vi "Untitled 1.vi"() -> ()   [LabVIEW 2026]
uses:
  CaptureJSONtypedef.ctl
  35900ef4-9114-49d9-b2d4-e1f00d13cbe6.vi
  <vilib>/JDP Science/JSONtext/JSON text to Variant.vi
  <vilib>/JDP Science/JSONtext/LVClass Serializer/JSONtext LVClass Serializer.lvclass
panel:
  out "Delta tMs":i32[](array[numeric])
  out "timingTicks64":string[](array[string])
  out "tMs":i32[](array[numeric])
  out "Index":i32[](array[numeric])
  out "Data out":T1
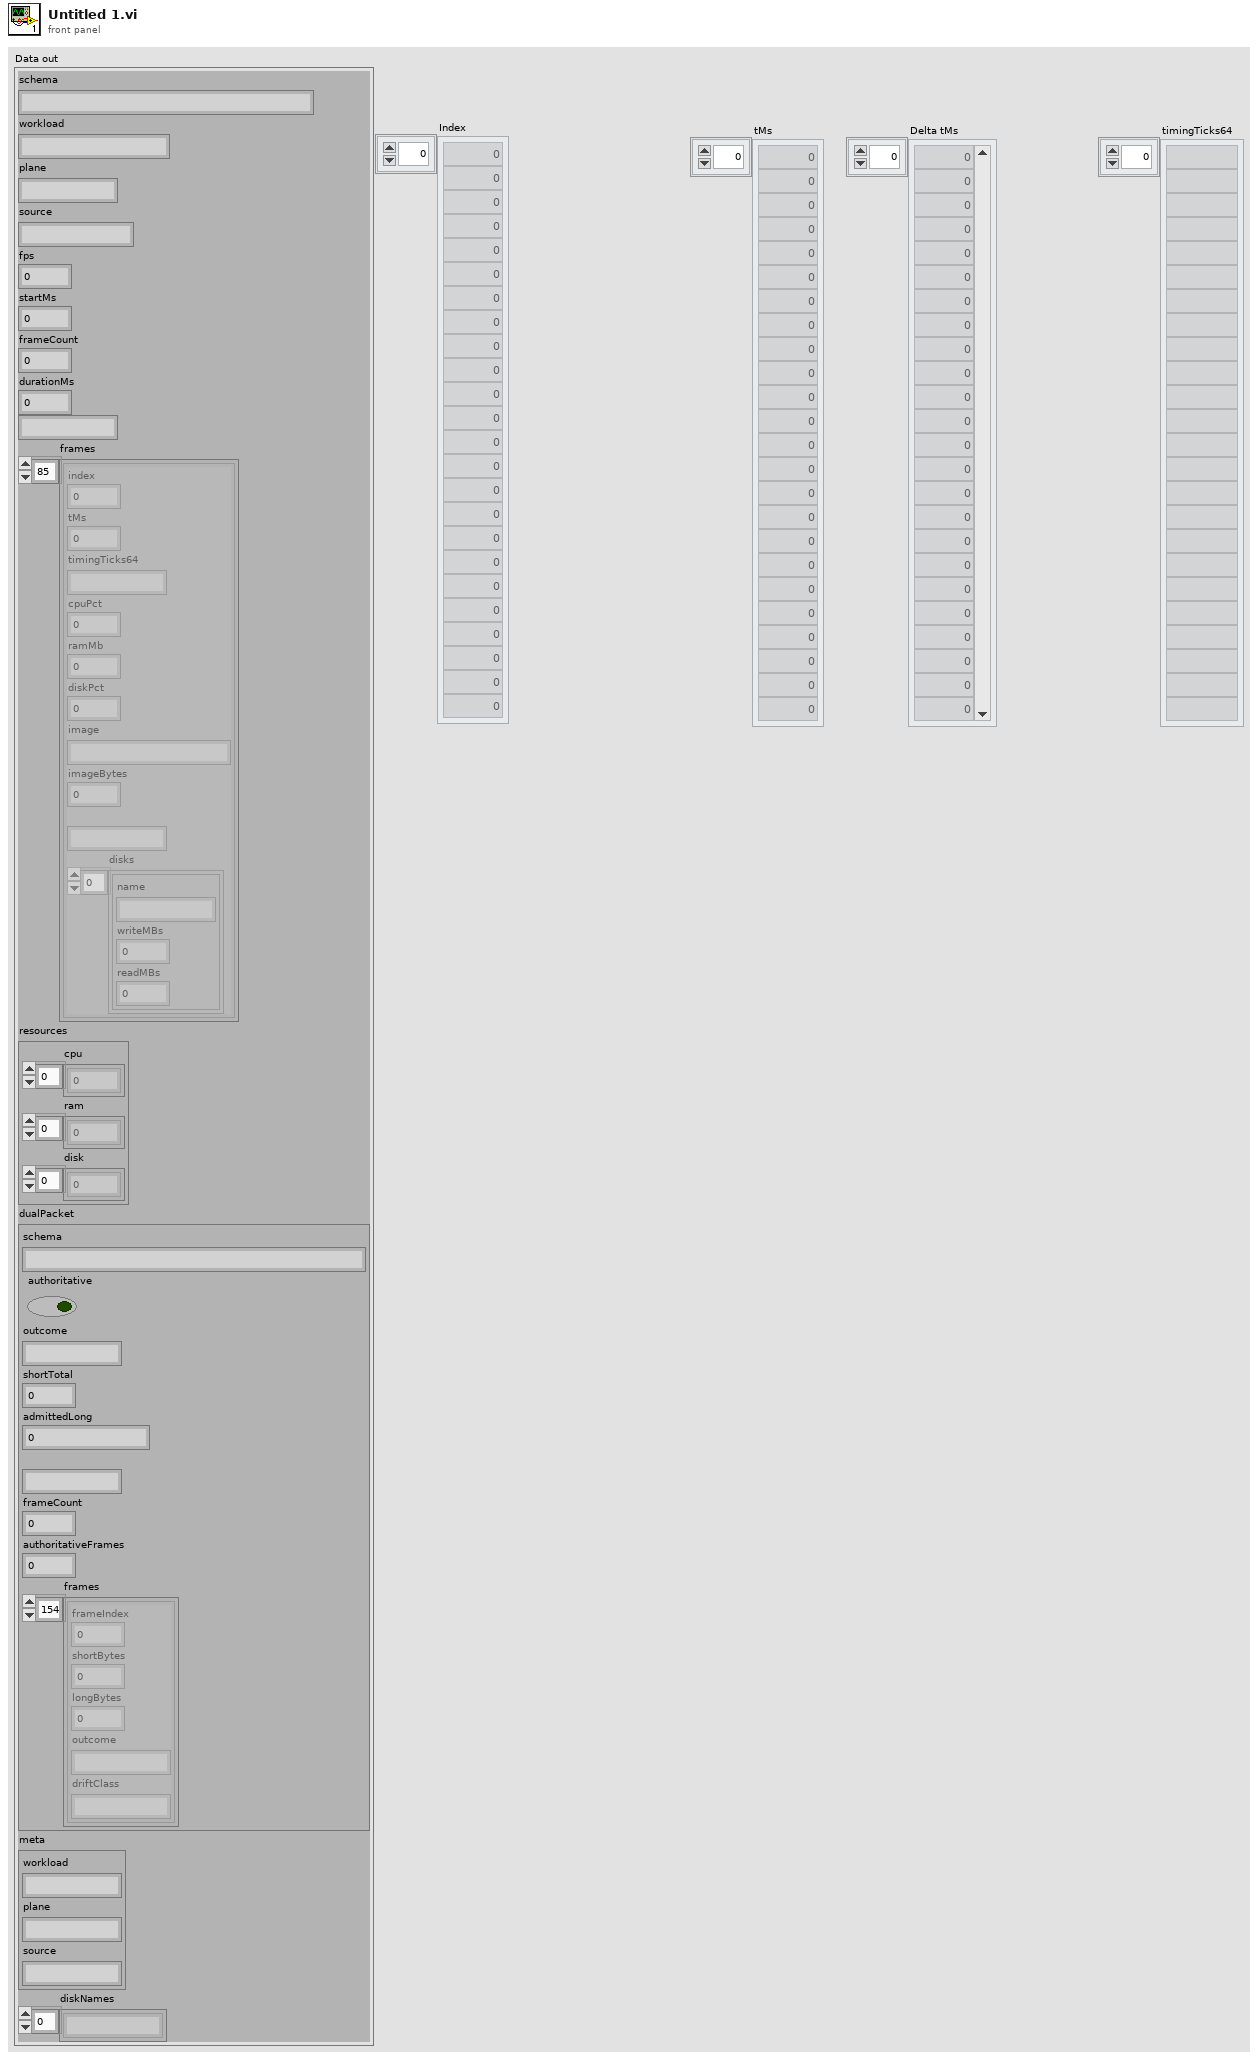
[diagram p1: front panel]
types:
  T1 = typedef "CaptureJSONtypedef.ctl" = cluster{"schema":string, "workload":string, "plane":string, "source":string, "fps":i32, "startMs":i32, "frameCount":i32, "durationMs":i32, string, "frames":cluster{"index":i32, "tMs":i32, "timingTicks64":string, "cpuPct":dbl, "ramMb":i32, "diskPct":dbl, "image":string, "imageBytes":i32, string, "disks":cluster{"name":string, "writeMBs":dbl, "readMBs":dbl}[]}[], "resources":cluster{"cpu":dbl[], "ram":dbl[], "disk":dbl[]}, "dualPacket":cluster{"schema":string, "authoritative":bool, "outcome":string, "shortTotal":i32, "admittedLong":i32, string, "frameCount":i32, "authoritativeFrames":i32, "frames":cluster{"frameIndex":i32, "shortBytes":i32, "longBytes":i32, "outcome":string, "driftClass":string}[]}, "meta":cluster{"workload":string, "plane":string, "source":string}, "diskNames":string[]}
  T2 = cluster{"index":i32, "tMs":i32, "timingTicks64":string, "cpuPct":dbl, "ramMb":i32, "diskPct":dbl, "image":string, "imageBytes":i32, string, "disks":cluster{"name":string, "writeMBs":dbl, "readMBs":dbl}[]}[]
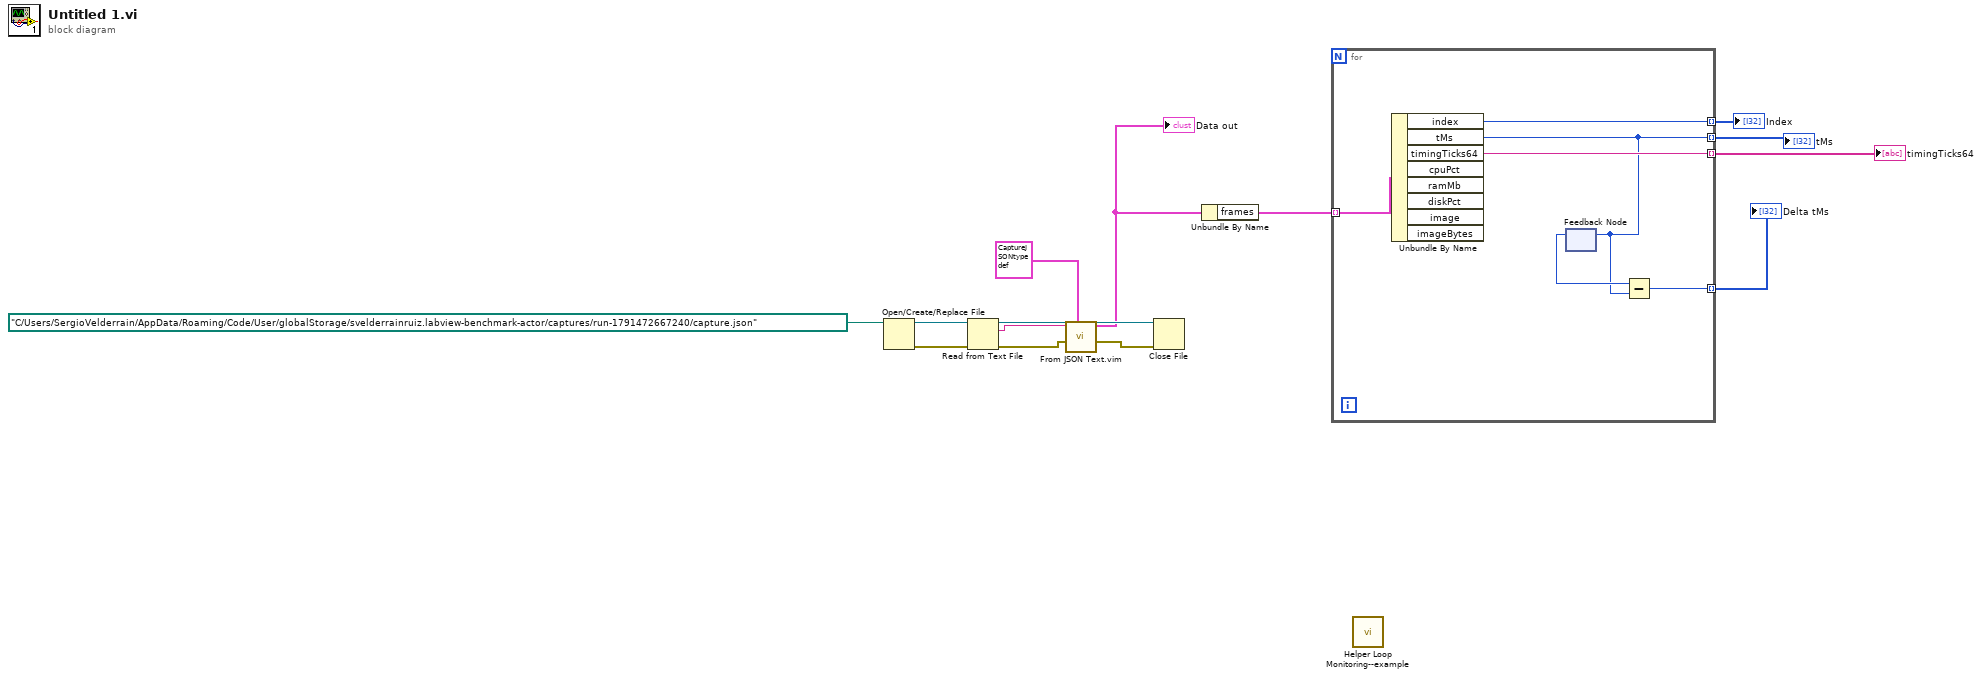
[diagram p0: block diagram]
diagram:
  n1 = Open/Create/Replace File(file path (use dialog)=path "C:/Users/SergioVelderrain/AppData/Roaming/Code/User/globalStorage/svelderrainruiz.labview-benchmark-actor/captures/run-1791472667240/capture.json") -> (refnum out=w13:refnum<file>, error out=w12:errorcluster)  [unwired: 5 in, 1 out]
  n2 = Read from Text File(file (use dialog)=w13, error in=w12) -> (refnum out=w14:refnum<file>, text=w8:string, error out=w10:errorcluster)  [unwired: 2 in, 1 out]
  n3 = call "From JSON Text.vim"("Data Type and Default Value"=T1 {"schema"="", "workload"="", "plane"="", "source"="", "fps"=0, "startMs"=0, "frameCount"=0, "durationMs"=0, "", "frames"=[], "resources"={"cpu"=[], "ram"=[], "disk"=[]}, "dualPacket"={"schema"="", "authoritative"=FALSE, "outcome"="", "shortTotal"=0, "admittedLong"=0, "", "frameCount"=0, "authoritativeFrames"=0, "frames"=[]}, "meta"={"workload"="", "plane"="", "source"=""}, "diskNames"=[]} ("CaptureJSONtypedef"), "error in (no error)"=w10, "JSON"=w8) -> ("error out"=w9:errorcluster, "Data out"=w6:T1)  [unwired: 7 in]
  "Data out" <- w6
  n4 = Close File(refnum=w14, error in=w9) -> ()  [unwired: 2 out]
  n5 = Unbundle By Name(w6) -> ("frames"=w5:T2)
  n6 = for {
    tunnel: w5 -> [w20] mode=indexing
    tunnel: [w19] -> w2 mode=indexing
    tunnel: [w16] -> w3 mode=indexing
    tunnel: [w18] -> w4 mode=indexing
    tunnel: [w15] -> w1 mode=indexing
    n7 = Unbundle By Name(w20) -> ("index"=w18:i32, "tMs"=w16:i32, "timingTicks64"=w19:string)  [unwired: 5 out]
    n8 = feedback-in #1(w16) -> ()
    n9 = feedback #1() -> (w17:i32)  [unwired: 1 in]
    n10 = Subtract(x=w17, y=w16) -> (x-y=w15:i32)
  }
  "Index" <- w4
  "tMs" <- w3
  "timingTicks64" <- w2
  "Delta tMs" <- w1
  n11 = call <vilib>:"Helper Loop Monitoring--example.vi"() -> ()  [unwired: 12 in]
